vi "AppendTimestamp.vi"(10 "String":string) -> (2 "String 2":string)   [LabVIEW 2013]
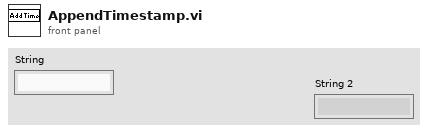
[diagram p1: front panel]
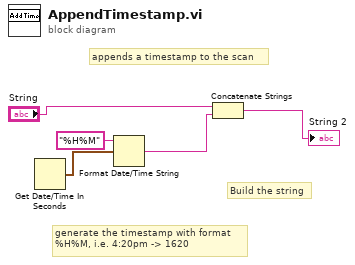
[diagram p0: block diagram]
diagram:
  # "Build the string"
  # "generate the timestamp with format\n%H%M, i.e. 4:20pm -> 1620"
  # "appends a timestamp to the scan"
  n1 = Get Date/Time In Seconds() -> (seconds since 1Jan1904=w5:timestamp)
  n2 = Format Date/Time String(time format string (%c)="%H%M", seconds (now)=w5) -> (date/time string=w2:string)  [unwired: 1 in]
  n3 = Concatenate Strings("String", w2) -> (→"String 2":string)
